vi "Read_ProcessConfig.vi"(8 "error in (no error)":errorcluster, 11 "Process in":refnum<class "Process.lvclass">) -> (0 "error out":errorcluster, 2 "ProcessConfig":T1={"Path"=path "", "Timeout"=0.0, "viInitString"="", "State"=enum."Closed"}, 3 "Process out":refnum<class "Process.lvclass">)   [LabVIEW 2013, in "Process.lvclass"]
uses:
  Process.lvclass
  050 - CONFIG/20 - ExternalProcesses/paramsExternalProcesses.ctl
  Process.lvclass/Process.ctl
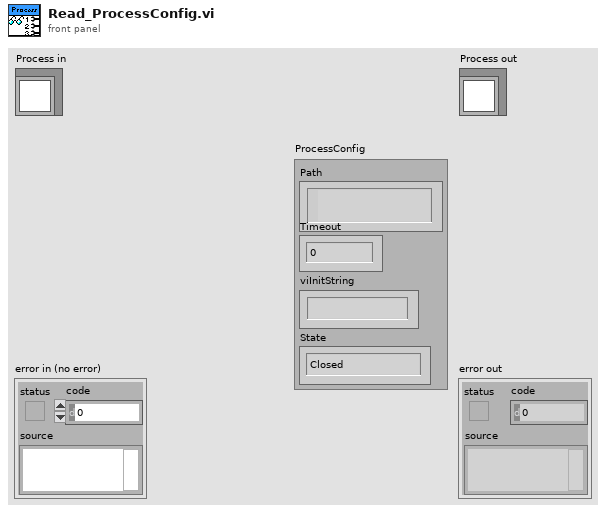
[diagram p1: front panel]
types:
  T1 = typedef "paramsExternalProcesses.ctl" = cluster{"Path":path, "Timeout":dbl, "viInitString":string, "State":enum32{"Invalid", "Standard", "Closed", "Hidden", "Minimized", "Maximized"}}
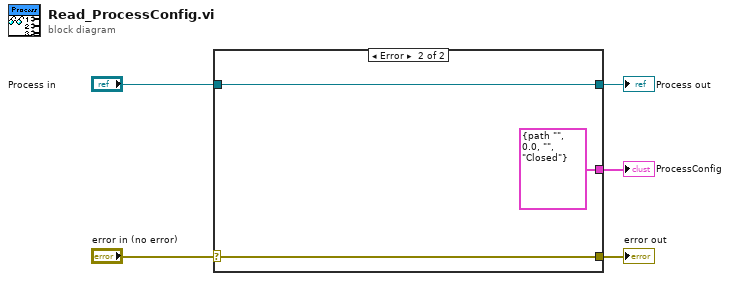
[diagram p0: block diagram]
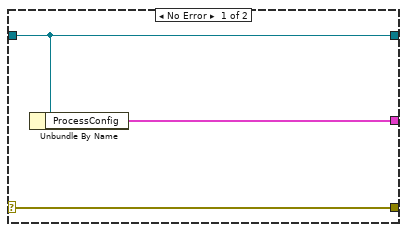
[diagram p2: hidden frame]
diagram:
  n1 = case shown="Error" "error in (no error)" {
    selector: "error in (no error)" -> [w8 w10]
    tunnel: [w8 w10] -> w4
    tunnel: [w7 w11] -> w2
    tunnel: "Process in" -> [w7 w11]
    tunnel: [w6 T1 {"Path"=path "", "Timeout"=0.0, "viInitString"="", "State"=enum."Closed"} ("ProcessConfig")] -> w1
    frame No Error {
      n2 = Unbundle By Name(w7) -> ("ProcessConfig"=w6:T1)
    }
    frame Error {
    }
  }
  "error out" <- w4
  "Process out" <- w2
  "ProcessConfig" <- w1
